vi "Vision Processing FGV.vi"(1 "New Vision Processing":string, 2 "Action":enum16{"Set", "Get"}(ring)=enum."Get") -> (0 "Vision Processing":string)   [LabVIEW 2016]
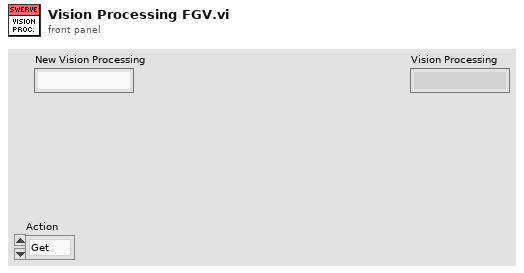
[diagram p1: front panel]
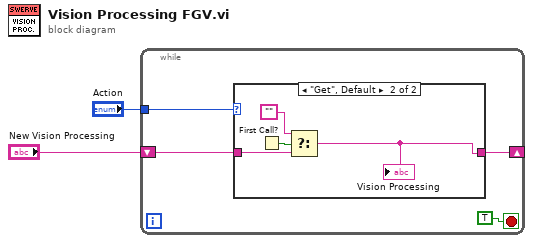
[diagram p0: block diagram]
diagram:
  n1 = while {
    shift-right: [w3] -> _
    shift-left: "New Vision Processing" -> [w4]
    tunnel: "Action" -> [w5]
    stop <- TRUE stop-if-true
    n2 = case shown="\"Get\", Default" w5 {
      tunnel: w4 -> [w7 w10]
      tunnel: [w7 w9] -> w3
      frame "Set" {
      }
      frame "Get", Default {
        n3 = First Call?() -> (First Call?: T/F=w11:bool)
        n4 = Select(t="", s=w11, f=w10) -> (s? t:f=w9:string)
        "Vision Processing" <- w9
      }
    }
  }
